vi "Configure.vi"(8 "error in (no error)":errorcluster, 10 "ConfigRef In":T1, 11 "Xitron in":refnum<class "Xitron.lvclass">) -> (0 "error out":errorcluster, 3 "Xitron out":refnum<class "Xitron.lvclass">)   [LabVIEW 2015, in "Xitron.lvclass"]
uses:
  Xitron.lvclass
  <vilib>/Utility/config.llb/Config Data RefNum.ctl
  Parent/Power Meter.lvclass/Power Meter.ctl
  Parent/Write Address.vi
  <vilib>/Utility/config.llb/Read Key (String).vi
  <vilib>/Utility/config.llb/NI_LVConfig.lvlib
panel:
  out "ConfigRef Out":T1
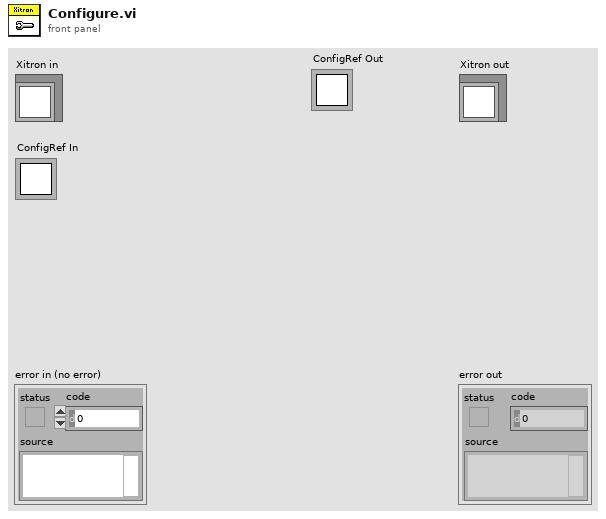
[diagram p1: front panel]
types:
  T1 = typedef "NI_LVConfig.lvlib/Config Data RefNum.ctl" = refnum<k1>
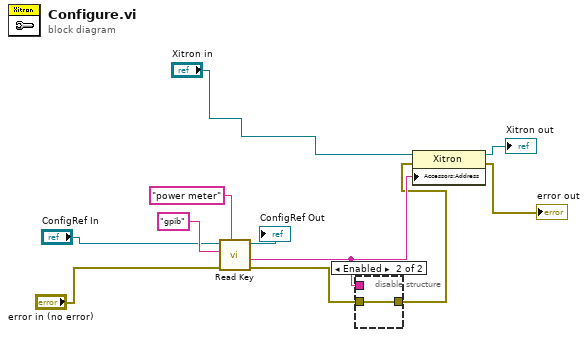
[diagram p0: block diagram]
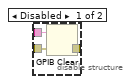
[diagram p2: hidden frame]
diagram:
  n1 = call-poly <vilib>:"Read Key.vi"("section"="power meter", "error in (no error)"="error in (no error)", "key"="gpib", "refnum"="ConfigRef In") -> ("error out"=w2:errorcluster, "value"=w3:string, "refnum out"=→"ConfigRef Out":T1)  [unwired: 4 in, 1 out]
  n2 = disable-structure shown="Enabled" {
    disable-tunnel: w3 -> [w14 _]
    disable-tunnel: w2 -> [w13 w15]
    disable-tunnel: [w12 w15] -> w1
    frame Disabled {
      n3 = GPIB Clear(2:w13, 3:w14) -> (0:w12:errorcluster)  [unwired: 1 out]
    }
    frame Enabled {
    }
  }
  n4 = property class="Xitron"(reference="Xitron in", error in=w1, "Accessors:Address"=w3) -> (reference out=→"Xitron out":refnum<class "Xitron.lvclass">, error out=→"error out":errorcluster)
